vi "Tell Init Self.vi"(7 "Actor in":refnum<class "Actor.lvclass">, 9 "Msg":T1 {"Teller"."Absolute Time" format="%<%x %.3X>T"}) -> (0 "Error out":errorcluster, 1 "Told":bool, 5 "Actor out":refnum<class "Actor.lvclass">)   [LabVIEW 2020, in "jettl.lvlib"]
uses:
  jettl.lvlib
  Actor/Actor.lvclass
  Msg Input/Msg Input.lvclass
  Msg Output/Msg Output.lvclass
  Msg/Msg.lvclass
  Unified Actor Relation.ctl
  Teller.ctl
  Msg.ctl
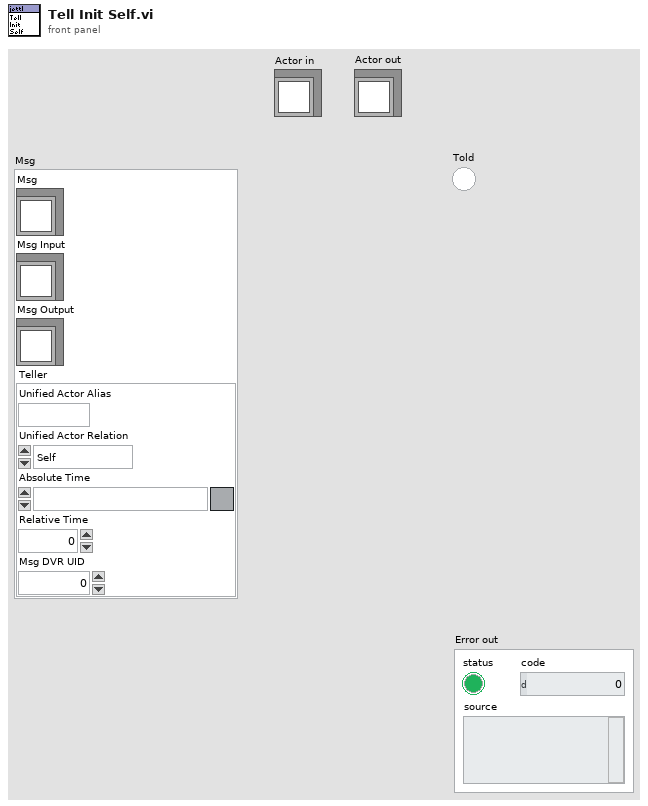
[diagram p1: front panel]
types:
  T1 = typedef "jettl.lvlib/Msg.ctl" = cluster{"Msg":refnum<class "Msg.lvclass">, "Msg Input":refnum<class "Msg Input.lvclass">, "Msg Output":refnum<class "Msg Output.lvclass">, "Teller":T2}
  T2 = typedef "jettl.lvlib/Teller.ctl" = cluster{"Unified Actor Alias":string, "Unified Actor Relation":T3, "Absolute Time":timestamp, "Relative Time":dbl, "Msg DVR UID":i32}
  T3 = typedef "jettl.lvlib/Unified Actor Relation.ctl" = enum16{"Self", "Parent", "Child"}
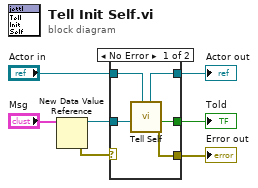
[diagram p0: block diagram]
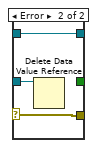
[diagram p2: hidden frame]
diagram:
  n1 = New Data Value Reference(data value="Msg") -> (data value reference=w7:refnum<data-value>, error out=w6:errorcluster)  [unwired: 1 in]
  n2 = case shown="No Error" w6 {
    selector: w6 -> [_ w15]
    tunnel: w7 -> [w12 w14]
    tunnel: [w11 w15] -> w1
    tunnel: "Actor in" -> [w10 w13]
    tunnel: [w9 w13] -> w3
    tunnel: [w8 _] -> w2
    frame No Error {
      n3 = call "Tell Self.vi"("Actor in"=w10, "Msg DVR"=w12) -> ("Error out"=w11:errorcluster, "Told"=w8:bool, "Actor out"=w9:refnum<class "Actor.lvclass">)  [unwired: 7 in]
    }
    frame Error {
      n4 = Delete Data Value Reference(data value reference=w14) -> ()  [unwired: 1 in, 2 out]
    }
  }
  "Error out" <- w1
  "Actor out" <- w3
  "Told" <- w2
